vi "Get Enqueuer.vi"(8 "error in (no error)":errorcluster, 11 "Output Actor Interface in":refnum<class "Output Actor Interface.lvclass">) -> (0 "error out":errorcluster, 2 "Actor Framework:Message Enqueuer":refnum<class "Message Enqueuer.lvclass">, 3 "Output Actor Interface out":refnum<class "Output Actor Interface.lvclass">)   [LabVIEW 2015, in "Output Actor Interface.lvclass"]
uses:
  Output Actor Interface.lvclass
  <vilib>/ActorFramework/Message Enqueuer/Message Enqueuer.lvclass
  Output Actor Interface.lvclass/Output Actor Interface.ctl
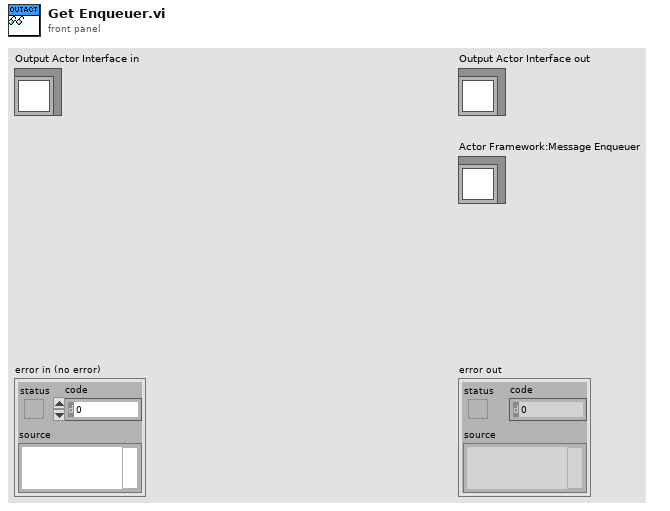
[diagram p1: front panel]
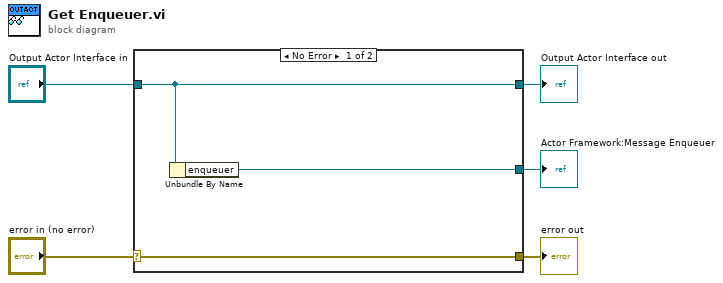
[diagram p0: block diagram]
diagram:
  n1 = case shown="No Error" "error in (no error)" {
    selector: "error in (no error)" -> [w8 w9]
    tunnel: [w8 w9] -> w4
    tunnel: [w7 w10] -> w2
    tunnel: "Output Actor Interface in" -> [w7 w10]
    tunnel: [w6 _] -> w1
    frame No Error {
      n2 = Unbundle By Name(w7) -> ("enqueuer"=w6:refnum<class "Message Enqueuer.lvclass">)
    }
    frame Error {
    }
  }
  "error out" <- w4
  "Output Actor Interface out" <- w2
  "Actor Framework:Message Enqueuer" <- w1
